vi "CleanConsole.vi"(11 "Console in":string) -> (3 "Console out":string)   [LabVIEW 2020]
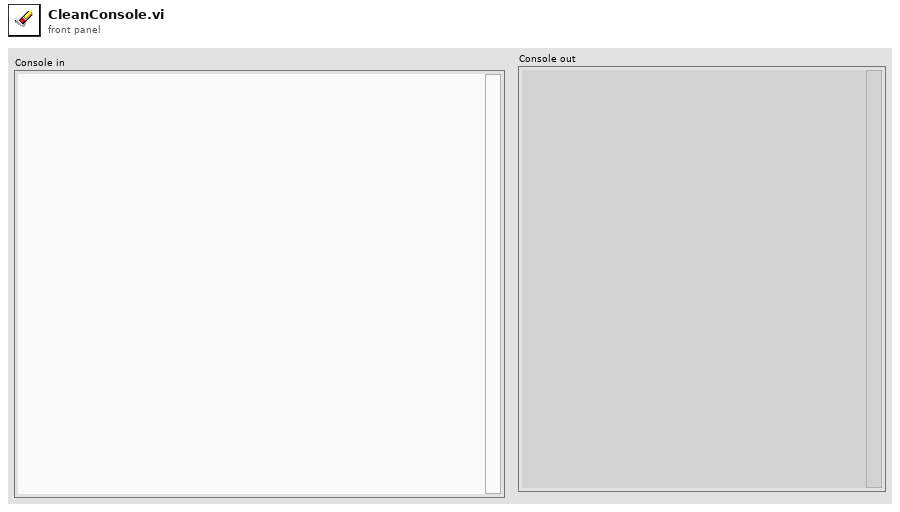
[diagram p1: front panel]
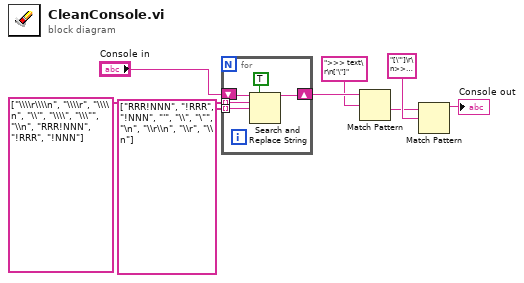
[diagram p0: block diagram]
diagram:
  n1 = for {
    tunnel: string[] ["\\\\r\\\\n", "\\\\r", "\\\\n", "\\'", "\\\\", "\\\"", "\\n", "RRR!NNN", "!RRR", "!NNN"] -> [w12] mode=indexing
    tunnel: string[] ["RRR!NNN", "!RRR", "!NNN", "'", "\\", "\"", "\n", "\\r\\n", "\\r", "\\n"] -> [w11] mode=indexing
    shift-right: [w10] -> w8
    shift-left: "Console in" -> [w9]
    n2 = Search and Replace String(replace all?=TRUE ("replace all? (F)"), input string=w9, search string=w12, replace string=w11) -> (result string=w10:string)  [unwired: 4 in, 3 out]
  }
  n3 = Match Pattern(string=w8, regular expression=">>> text\r\n['\"]" ("replace string (\"\")")) -> (after substring=w2:string)  [unwired: 1 in, 3 out]
  n4 = Match Pattern(string=w2, regular expression="[\"']\r\n>>> " ("replace string (\"\")")) -> (before substring=→"Console out":string)  [unwired: 1 in, 3 out]
